vi "XY Graph Graph Axes Chooser Dialog.vi"(8 "Error In":errorcluster, 11 "XYGraph Ref":refnum<vi>) -> (0 "Error Out":errorcluster, 1 "Message":string, 2 "Cancelled":bool, 3 "XYGraph Ref dup":refnum<vi>)   [LabVIEW 2019, in "XY Graph Add-Ons.lvlib"]
uses:
  XY Graph Add-Ons.lvlib
panel:
  out "Y Scale":i32
  out "X Scale":i32
  in  "Y Axes":i32(listbox)
  in  "X Axes":i32(listbox)
  in  "Cancel":bool
  in  "OK":bool
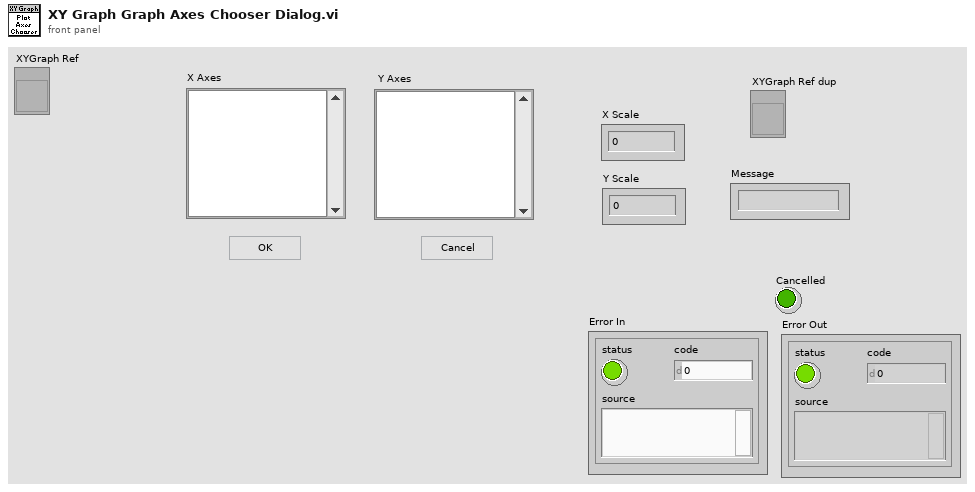
[diagram p1: front panel]
types:
  T1 = typedef "XY Graph Add-Ons.lvlib/XY Graph Refnum.ctl" = refnum<vi>
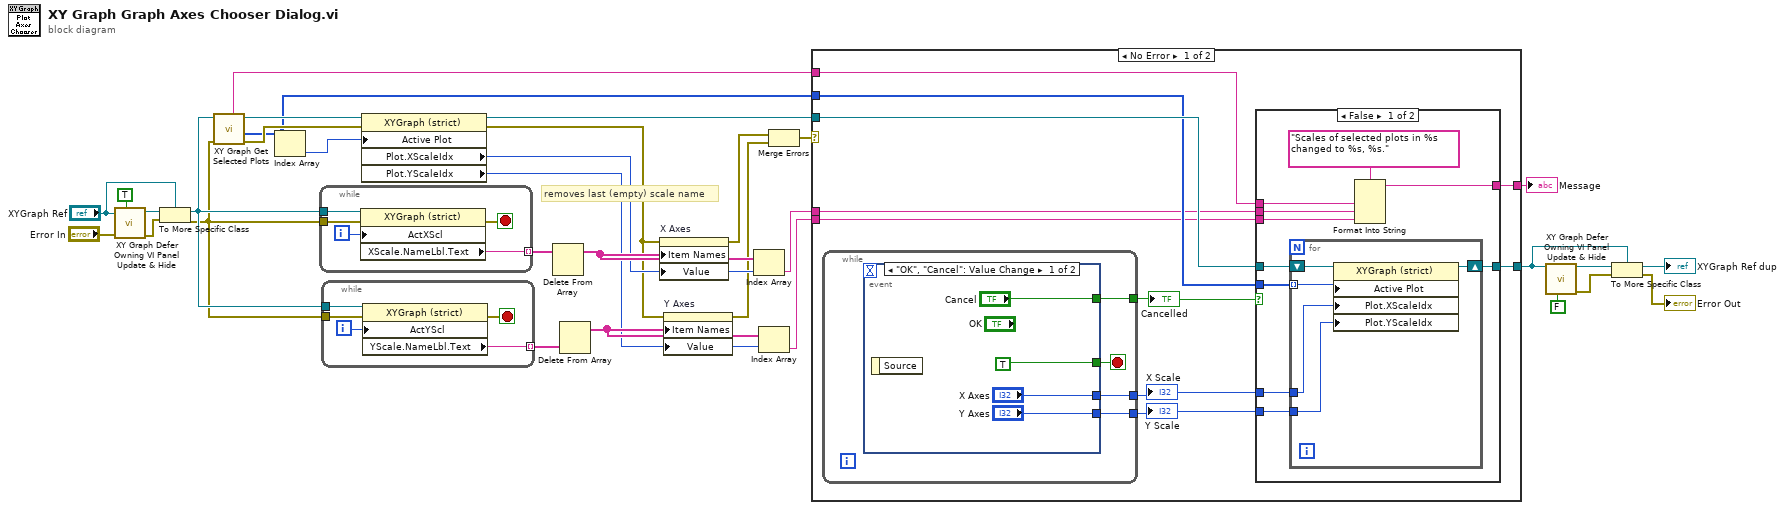
[diagram p0: block diagram]
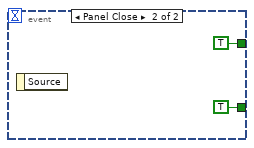
[diagram p3: hidden frame]
diagram:
  # "removes last (empty) scale name"
  n1 = call "XY Graph Defer Owning VI Panel Update & Hide.vi"("Defer Owning Panel Update"=TRUE, "error in (no error)"="Error In", "XY Graph Refnum in"="XYGraph Ref") -> ("error out"=w16:errorcluster, "XY Graph Refnum out"=w14:refnum<vi>)  [unwired: 7 in]
  n2 = To More Specific Class(target class="XYGraph Ref", reference=w14, error in=w16) -> (specific class reference=w12:refnum<vi>, error out=w11:errorcluster)
  n3 = call "XY Graph Get Selected Plots.vi"("error in (no error)"=w11, "XYGraph in"=w12) -> ("error out"=w29:errorcluster, "Selected Plots"=w26:i32[], "XYGraph out"=w30:T1, "Graph Caption"=w25:string)  [unwired: 5 in, 1 out]
  n4 = Index Array(array=w26) -> (element=w28:i32)  [unwired: 1 in]
  n5 = while {
    tunnel: w12 -> [w37]
    tunnel: [w34] -> w32 mode=indexing
    tunnel: w11 -> [w33]
    i -> [w36]
    stop <- w35 stop-if-true
    n6 = property class="XYGraph (strict)"(reference=w37, error in=w33, "ActXScl"=w36) -> (error out=w35:errorcluster, "XScale.NameLbl.Text"=w34:string)  [unwired: 1 out]
  }
  n7 = while {
    tunnel: w12 -> [w42]
    tunnel: [w39] -> w31 mode=indexing
    tunnel: w11 -> [w38]
    i -> [w41]
    stop <- w40 stop-if-true
    n8 = property class="XYGraph (strict)"(reference=w42, error in=w38, "ActYScl"=w41) -> (error out=w40:errorcluster, "YScale.NameLbl.Text"=w39:string)  [unwired: 1 out]
  }
  n9 = property class="XYGraph (strict)"(reference=w30, error in=w29, "Active Plot"=w28) -> (reference out=w27:T1, error out=w5:errorcluster, "Plot.XScaleIdx"=w22:u32, "Plot.YScaleIdx"=w20:u32)
  n10 = Delete From Array(array=w32) -> (array with subset deleted=w23:string[])  [unwired: 2 in, 1 out]
  n11 = Delete From Array(array=w31) -> (array with subset deleted=w21:string[])  [unwired: 2 in, 1 out]
  n12 = property on="X Axes" class="LstBox (strict)"(error in=w5, "Item Names"=w23, "Value"=w22) -> (error out=w4:errorcluster)  [unwired: 1 in, 1 out]
  n13 = property on="Y Axes" class="LstBox (strict)"(error in=w5, "Item Names"=w21, "Value"=w20) -> (error out=w3:errorcluster)  [unwired: 1 in, 1 out]
  n14 = Index Array(array=w23, index=w22) -> (element=w19:string)
  n15 = Index Array(array=w21, index=w20) -> (element=w18:string)
  n16 = Merge Errors(w4, w3) -> (w2:errorcluster)
  n17 = case shown="No Error" w2 {
    tunnel: w27 -> [w51 w79]
    tunnel: w26 -> [w50 _]
    tunnel: w25 -> [w47 _]
    tunnel: [w46 _] -> w24
    tunnel: w19 -> [w45 _]
    tunnel: w18 -> [w44 _]
    tunnel: [w43 w79] -> w10
    frame No Error {
      n18 = while {
        tunnel: [w71] -> w52
        tunnel: [w70] -> w49
        tunnel: [w69] -> w48
        stop <- w72 stop-if-true
        n19 = event shown="[0] \"OK\", \"Cancel\": Value Change" {
          selector: _ -> [_ _]
          dyn-events: _ -> [_ _]
          timeout: _ -> [_ _]
          tunnel: [TRUE TRUE] -> w72
          tunnel: ["Cancel" TRUE ("Cancel")] -> w71
          tunnel: ["X Axes" _] -> w70
          tunnel: ["Y Axes" _] -> w69
          event "OK", "Cancel": Value Change {
            n20 = event-data() -> ()  [unwired: 1 in, 1 out]
          }
          event Panel Close {
            n21 = event-data() -> ()  [unwired: 1 in, 1 out]
          }
        }
      }
      "Cancelled" <- w52
      "X Scale" <- w49
      "Y Scale" <- w48
      n22 = case shown="False" w52 {
        tunnel: w51 -> [w62 w68]
        tunnel: w50 -> [w61 _]
        tunnel: w49 -> [w60 _]
        tunnel: w48 -> [w59 _]
        tunnel: w47 -> [w58 _]
        tunnel: [w56 _] -> w46
        tunnel: w45 -> [w55 _]
        tunnel: w44 -> [w54 _]
        tunnel: [w53 w68] -> w43
        frame False {
          n23 = for {
            tunnel: w61 -> [w66] mode=indexing
            tunnel: w60 -> [w65]
            tunnel: w59 -> [w64]
            shift-right: [w63] -> w53
            shift-left: w62 -> [w67]
            n24 = property class="XYGraph (strict)"(reference=w67, "Active Plot"=w66, "Plot.XScaleIdx"=w65, "Plot.YScaleIdx"=w64) -> (reference out=w63:T1)  [unwired: 1 in, 1 out]
          }
          n25 = Format Into String(format string="Scales of selected plots in %s changed to %s, %s.", w58, w55, w54) -> (resulting string=w56:string)  [unwired: 2 in, 1 out]
        }
        frame True {
        }
      }
    }
    frame Error {
    }
  }
  "Message" <- w24
  n26 = call "XY Graph Defer Owning VI Panel Update & Hide.vi"("Defer Owning Panel Update"=FALSE, "XY Graph Refnum in"=w10) -> ("error out"=w8:errorcluster, "XY Graph Refnum out"=w9:refnum<vi>)  [unwired: 8 in]
  n27 = To More Specific Class(target class=w10, reference=w9, error in=w8) -> (specific class reference=→"XYGraph Ref dup":T1, error out=→"Error Out":errorcluster)
